vi "ToggleCursor.vi"(8 "error in (no error)":errorcluster, 11 "Show":bool) -> (0 "error out":errorcluster)   [LabVIEW 2015]
uses:
  User32.dll
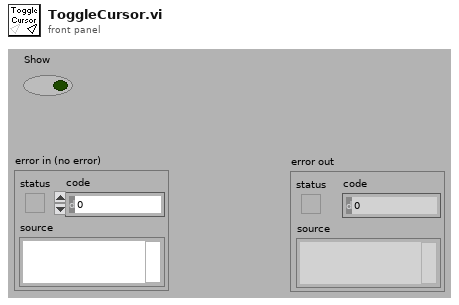
[diagram p1: front panel]
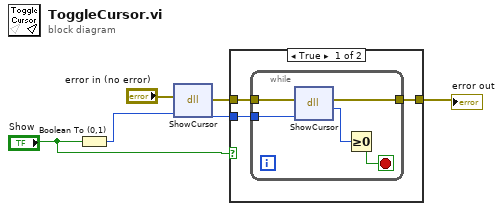
[diagram p0: block diagram]
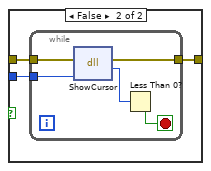
[diagram p2: hidden frame]
diagram:
  n1 = Boolean To (0,1)(Boolean="Show") -> (0, 1=w5:i16)
  n2 = dll-call lib="User32.dll" fn="ShowCursor"(error in="error in (no error)", "bShow"=w5) -> (error out=w2:errorcluster, "bShow"=w3:u8)  [unwired: 2 in, 2 out]
  n3 = case shown="True" "Show" {
    tunnel: w3 -> [w9 w17]
    tunnel: w2 -> [w8 w16]
    tunnel: [w7 w15] -> w1
    frame True {
      n4 = while {
        tunnel: w9 -> [w13]
        tunnel: w8 -> [w11]
        tunnel: [w10] -> w7
        stop <- w14 stop-if-true
        n5 = dll-call lib="User32.dll" fn="ShowCursor"(error in=w11, "bShow"=w13) -> (error out=w10:errorcluster, "dispCounter"=w12:i32)  [unwired: 3 in, 1 out]
        n6 = Greater Or Equal To 0?(x=w12) -> (x >= 0?=w14:bool)
      }
    }
    frame False {
      n7 = while {
        tunnel: w17 -> [w21]
        tunnel: w16 -> [w19]
        tunnel: [w18] -> w15
        stop <- w22 stop-if-true
        n8 = dll-call lib="User32.dll" fn="ShowCursor"(error in=w19, "bShow"=w21) -> (error out=w18:errorcluster, "dispCounter"=w20:i32)  [unwired: 3 in, 1 out]
        n9 = Less Than 0?(x=w20) -> (x < 0?=w22:bool)
      }
    }
  }
  "error out" <- w1
